vi "Read XY graph ref.vi"(8 "error in (no error)":errorcluster, 10 "Combo Box":string(combo)="Kinetics", 11 "Control-Client in":refnum<class "Control-Client.lvclass">) -> (0 "error out":errorcluster, 2 "XY graph ref":refnum<vi>, 3 "Control-Client out":refnum<class "Control-Client.lvclass">)   [LabVIEW 2020, in "Control-Client.lvclass"]
uses:
  Control-Client.lvclass
  Control-Client.lvclass/Control-Client.ctl
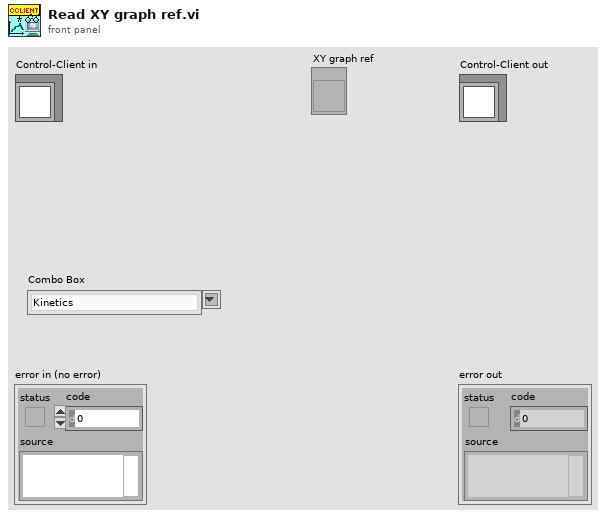
[diagram p1: front panel]
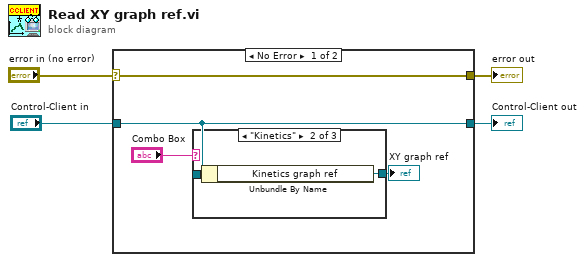
[diagram p0: block diagram]
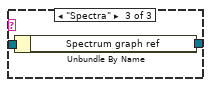
[diagram p3: hidden frame]
diagram:
  n1 = case shown="No Error" "error in (no error)" {
    selector: "error in (no error)" -> [w8 w13]
    tunnel: [w8 w13] -> w3
    tunnel: [w6 w14] -> w1
    tunnel: "Control-Client in" -> [w6 w14]
    frame No Error {
      n2 = case shown="\"Kinetics\"" "Combo Box" {
        tunnel: w6 -> [_ w10 w12]
        tunnel: [_ w9 w11] -> w5
        frame "False", Default {
        }
        frame "Kinetics" {
          n3 = Unbundle By Name(w10) -> ("Kinetics graph ref"=w9:refnum<vi>)
        }
        frame "Spectra" {
          n4 = Unbundle By Name(w12) -> ("Spectrum graph ref"=w11:refnum<vi>)
        }
      }
      "XY graph ref" <- w5
    }
    frame Error {
    }
  }
  "error out" <- w3
  "Control-Client out" <- w1
